vi "Calculate Scan Time.vi"(7 "Step Sizes":sgl[](array[numeric]), 8 "Scan Mode":enum16{"Raster", "Serpentine"}(ring), 9 "Speed Control (mm/s)":sgl=1.0 min=0.1, 10 "Line Count":i32=6 caption="Y Pixels", 11 "Pixel Count":i32=6 caption="X Pixels") -> (0 "Seconds":u8, 1 "Mins":u8, 2 "Hours":u8, 3 "TimeString":string, 4 "total time (sec)":sgl)   [LabVIEW 2020]
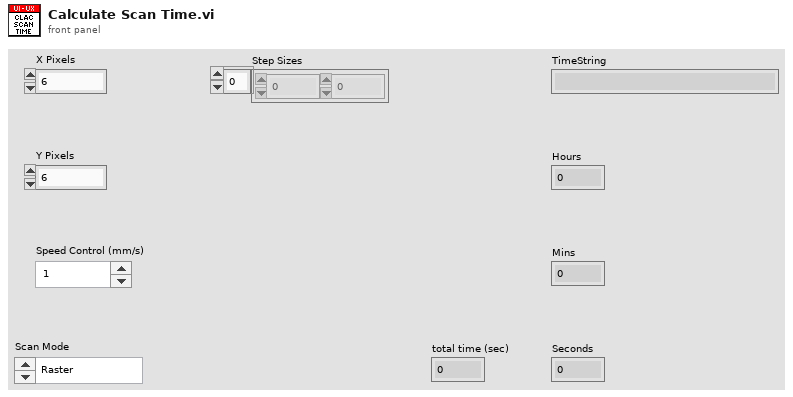
[diagram p1: front panel]
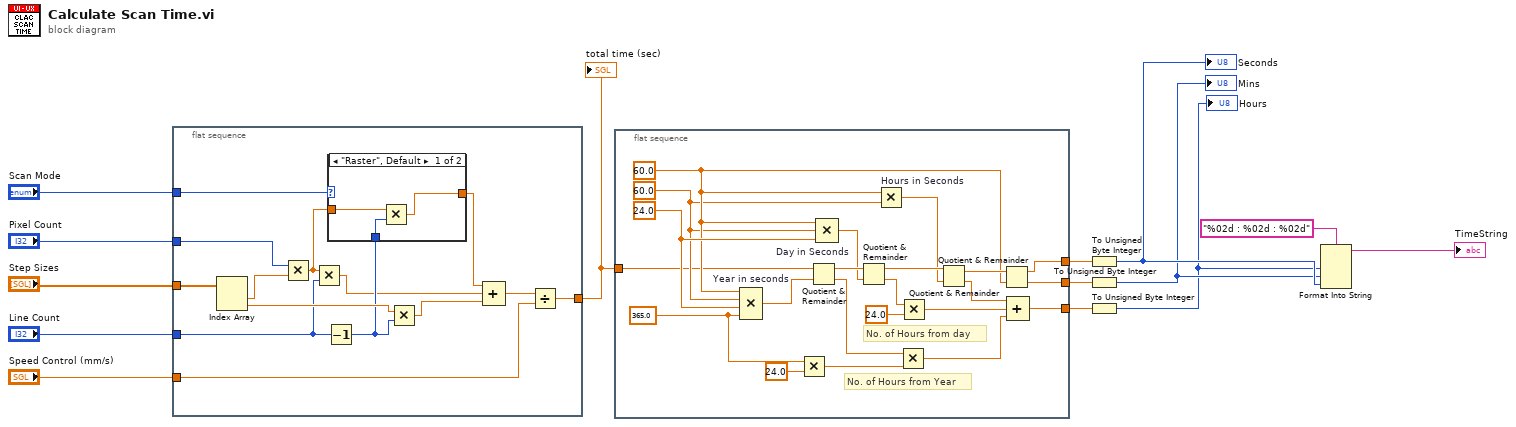
[diagram p0: block diagram]
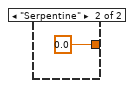
[diagram p2: hidden frame]
diagram:
  n1 = flat-sequence {
    tunnel: "Step Sizes" -> [w28]
    tunnel: "Pixel Count" -> [w27]
    tunnel: "Line Count" -> [w24]
    tunnel: "Speed Control (mm/s)" -> [w23]
    tunnel: "Scan Mode" -> [w19]
    tunnel: [w17] -> w9
    frame #0 {
      n2 = Index Array(array=w28) -> (element #1=w26:sgl, element #2=w25:sgl)  [unwired: 2 in]
      n3 = Multiply(x=w27, y=w26) -> (x*y=w22:sgl)
      n4 = Multiply(x=w22, y=w24) -> (x*y=w15:sgl)
      n5 = Decrement(x=w24) -> (x-1=w21:i32)
      n6 = case shown="\"Raster\", Default" w19 {
        tunnel: w22 -> [w31 _]
        tunnel: w21 -> [w30 _]
        tunnel: [w29 sgl 0.0] -> w18
        frame "Raster", Default {
          n7 = Multiply(x=w31, y=w30) -> (x*y=w29:sgl)
        }
        frame "Serpentine" {
        }
      }
      n8 = Multiply(x=w25, y=w21) -> (x*y=w16:sgl)
      n9 = Compound Arithmetic op=ADD(w18, w15, w16) -> (w20:sgl)
      n10 = Divide(x=w20, y=w23) -> (x/y=w17:sgl)
    }
  }
  n11 = flat-sequence {
    tunnel: [w42] -> w7
    tunnel: [w41] -> w6
    tunnel: [w40] -> w5
    tunnel: w9 -> [w33]
    frame #0 {
      w36 = 365.0
      w48 = 24.0
      w38 = 60.0
      w39 = 60.0
      # "No. of Hours from day"
      # "No. of Hours from Year"
      n12 = Compound Arithmetic op=MULTIPLY "Year in seconds"(w39, w38, w48, w36) -> (w54:dbl)
      n13 = Multiply(x=w36, y=24.0) -> (x*y=w34:dbl)
      n14 = Quotient & Remainder(x=w33, y=w54) -> (x-y*floor(x/y)=w53:dbl, floor(x/y)=w50:dbl)
      n15 = Compound Arithmetic op=MULTIPLY "Day in Seconds"(w39, w38, w48) -> (w49:dbl)
      n16 = Quotient & Remainder(x=w53, y=w49) -> (x-y*floor(x/y)=w52:dbl, floor(x/y)=w47:dbl)
      n17 = Multiply "Hours in Seconds"(x=w39, y=w38) -> (x*y=w51:dbl)
      n18 = Multiply(x=w50, y=w34) -> (x*y=w43:dbl)
      n19 = Multiply(x=w47, y=24.0) -> (x*y=w44:dbl)
      n20 = Quotient & Remainder(x=w52, y=w51) -> (x-y*floor(x/y)=w46:dbl, floor(x/y)=w45:dbl)
      n21 = Quotient & Remainder(x=w46, y=w39) -> (x-y*floor(x/y)=w40:dbl, floor(x/y)=w41:dbl)
      n22 = Compound Arithmetic op=ADD(w45, w44, w43) -> (w42:dbl)
    }
  }
  n23 = To Unsigned Byte Integer(number=w5) -> (unsigned 8bit integer=w3:u8)
  "Seconds" <- w3
  n24 = To Unsigned Byte Integer(number=w6) -> (unsigned 8bit integer=w2:u8)
  "Mins" <- w2
  n25 = To Unsigned Byte Integer(number=w7) -> (unsigned 8bit integer=w1:u8)
  "Hours" <- w1
  n26 = Format Into String(format string="%02d : %02d : %02d", w1, w2, w3) -> (resulting string=→"TimeString":string)  [unwired: 2 in, 1 out]
  "total time (sec)" <- w9
